vi "ECOG-Apply Filter.vi"(0 "display in":T1 {"IIR Filter"."Forward Coefficients" format="%.4f"; "IIR Filter"."Reverse Coefficients" format="%.4f"}, 5 "Filter?":bool, 7 "new data":dbl[](array[numeric])) -> (4 "display out":T1 {"IIR Filter"."Forward Coefficients" format="%.4f"; "IIR Filter"."Reverse Coefficients" format="%.4f"}, 8 "Filtered X":dbl[](array[numeric]))   [LabVIEW 2020]
uses:
  Typedefs/ECOG-Display.ctl
  <vilib>/Analysis/3filter.llb/IIR Cascade Filter with I.C. (DBL).vi
  <vilib>/Analysis/NI_AALBase.lvlib
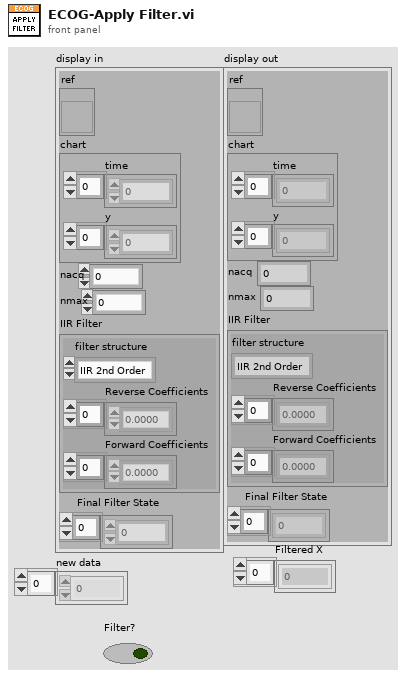
[diagram p1: front panel]
types:
  T1 = typedef "ECOG-Display.ctl" = cluster{"ref":refnum<vi>, "chart":cluster{"time":dbl[], "y":dbl[]}, "nacq":i32, "nmax":i32, "IIR Filter":cluster{"filter structure":enum32{"IIR 2nd Order", "IIR 4th Order"}, "Reverse Coefficients":dbl[], "Forward Coefficients":dbl[]}, "Final Filter State":dbl[]}
  T2 = cluster{"filter structure":enum32{"IIR 2nd Order", "IIR 4th Order"}, "Reverse Coefficients":dbl[], "Forward Coefficients":dbl[]}
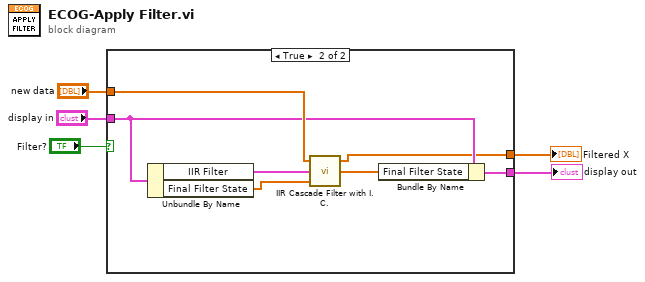
[diagram p0: block diagram]
diagram:
  n1 = case shown="True" "Filter?" {
    tunnel: "new data" -> [w6 w13]
    tunnel: "display in" -> [w7 w11]
    tunnel: [w6 w9] -> w3
    tunnel: [w7 w8] -> w2
    frame False {
    }
    frame True {
      n2 = Unbundle By Name(w11) -> ("IIR Filter"=w14:T2, "Final Filter State"=w12:dbl[])
      n3 = call-poly <vilib>:"IIR Cascade Filter with I.C..vi"("Initial Filter State"=w12, "IIR Filter Cluster"=w14, "X"=w13) -> ("Final Filter State"=w10:dbl[], "Filtered X"=w9:dbl[])  [unwired: 1 out]
      n4 = Bundle By Name(cluster=w11, "Final Filter State"=w10) -> (w8:T1)
    }
  }
  "display out" <- w2
  "Filtered X" <- w3
